vi "CreateSystemReference.vi"(8 "error in (no error)":errorcluster, 9 "Pane":refnum<vi>, 10 "ThisVIReference":refnum<vi>) -> (0 "error out":errorcluster, 1 "CommandQueueOut":refnum<queue>, 2 "DataNotifierOut":refnum<notifier>, 3 "ControlValueChangeEventRef":refnum<event-registration>)   [LabVIEW 2013]
uses:
  SystemData.lvclass/SystemData.lvclass
  RootCommand.lvclass/RootCommand.lvclass
  <vilib>/Utility/miscctls.llb/LVPointTypeDef.ctl
  Initialize.lvclass/Initialize.lvclass
  SystemData.lvclass/SystemData.lvclass/SystemData.ctl
  Generator.lvclass/Generator.lvclass
panel:
  # "建立系統運行參考"
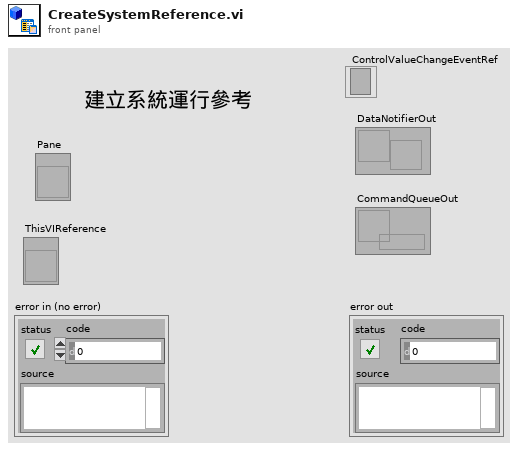
[diagram p1: front panel]
types:
  T1 = typedef "LVPointTypeDef.ctl" = cluster{"Horizontal":i16, "Vertical":i16}
  T2 = typedef "SystemData.lvclass/SystemDataTypeDefine.ctl" = cluster{"ThisVIParameter":cluster{"ThisVIPath":path, "ThisVIReference":refnum<vi>, "AllControlReference":refnum<vi>[]}, "GeneratorParameter":cluster{"Frequency":dbl, "Amplitude":dbl}, "WaveformBuffer":waveform(dbl), "SourceSelect":u16, "GeneratorClassArray":refnum<class "Generator.lvclass">[]}
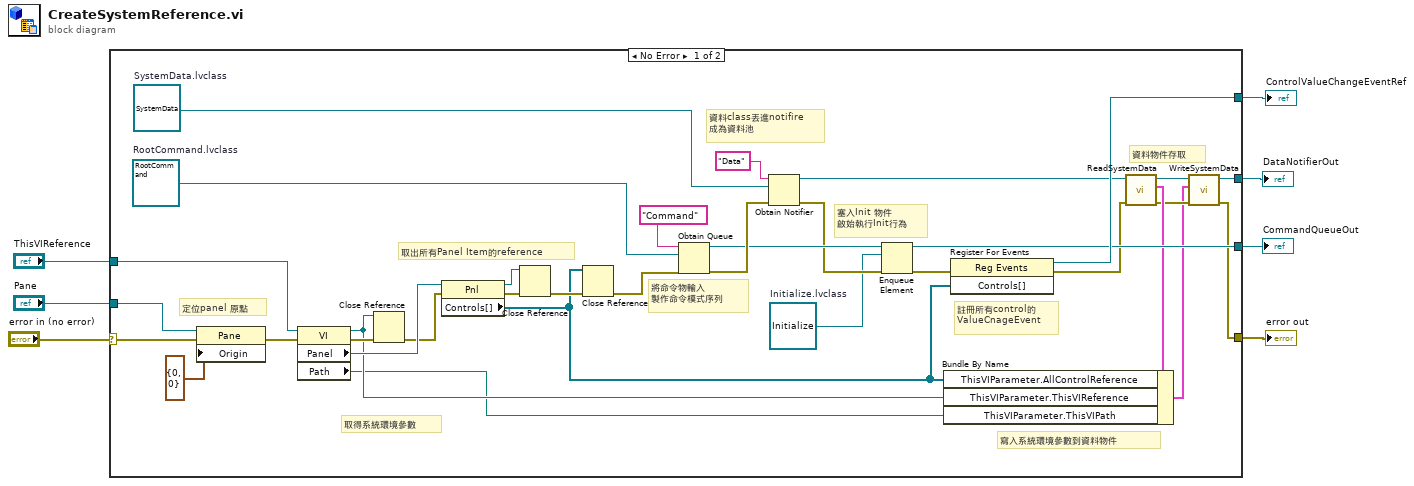
[diagram p0: block diagram]
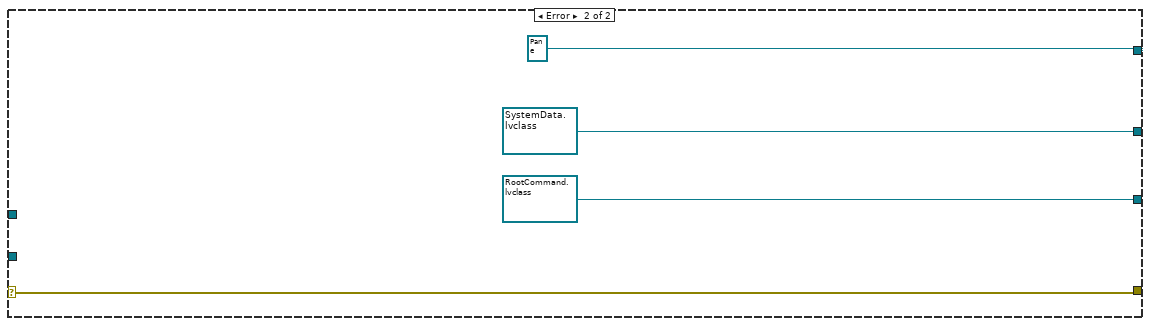
[diagram p2: hidden frame]
diagram:
  n1 = case shown="No Error" "error in (no error)" {
    selector: "error in (no error)" -> [w16 w45]
    tunnel: [w41 refnum<event-registration> refnum ("Event Registration Refnum")] -> w7
    tunnel: [w27 refnum<notifier> refnum ("DataNotifierOut")] -> w2
    tunnel: [w36 refnum<queue> refnum ("queue out")] -> w1
    tunnel: [w23 w45] -> w6
    tunnel: "ThisVIReference" -> [w29 _]
    tunnel: "Pane" -> [w15 _]
    frame No Error {
      w10 = refnum<class "Initialize.lvclass"> refnum  # Initialize.lvclass
      w20 = refnum<class "SystemData.lvclass"> refnum  # SystemData.lvclass
      w19 = refnum<class "RootCommand.lvclass"> refnum  # RootCommand.lvclass
      # "定位panel 原點"
      # "資料物件存取"
      # "塞入Init 物件\n啟始執行Init行為"
      # "取出所有Panel Item的reference"
      # "取得系統環境參數"
      # "寫入系統環境參數到資料物件"
      # "註冊所有control的\nValueCnageEvent"
      # "資料class丟進notifire\n成為資料池"
      # "將命令物輸入\n製作命令模式序列"
      n2 = property class="Pane"(reference=w15, error in=w16, "Origin"=T1 {"Horizontal"=0, "Vertical"=0}) -> (error out=w17:errorcluster)  [unwired: 1 out]
      n3 = property class="VI"(reference=w29, error in=w17) -> (reference out=w22:refnum<vi>, error out=w30:errorcluster, "Panel"=w31:refnum<vi>, "Path"=w21:path)
      n4 = Close Reference(reference=w22, error in (no error)=w30) -> (error out=w18:errorcluster)
      n5 = property class="Pnl"(reference=w31, error in=w18) -> (reference out=w33:refnum<vi>, error out=w32:errorcluster, "Controls[]"=w8:refnum<vi>[])
      n6 = Close Reference(reference=w33, error in (no error)=w32) -> (error out=w9:errorcluster)
      n7 = Close Reference(reference=w8, error in (no error)=w9) -> (error out=w11:errorcluster)
      n8 = Obtain Queue(name (unnamed)="Command", element data type=w19, error in (no error)=w11) -> (queue out=w37:refnum<queue>, error out=w40:errorcluster)  [unwired: 2 in, 1 out]
      n9 = Obtain Notifier(name (unnamed)="Data", notification data type=w20, error in (no error)=w40) -> (notifier out=w12:refnum<notifier>, error out=w35:errorcluster)  [unwired: 1 in, 1 out]
      n10 = Enqueue Element(queue=w37, element=w10, error in (no error)=w35) -> (queue out=w36:refnum<queue>, error out=w34:errorcluster)  [unwired: 1 in, 1 out]
      n11 = register-events(error in=w34, w8) -> (reference out=w41:refnum<event-registration>, error out=w26:errorcluster)  [unwired: 1 in]
      n12 = call "ReadSystemData.vi"("error in (no error)"=w26, "DataNotifierIn"=w12) -> ("error out"=w24:errorcluster, "SystemData"=w25:T2, "DataNotifierIn"=w28:refnum<notifier>)  [unwired: 7 in]
      n13 = Bundle By Name(cluster=w25, "ThisVIParameter.AllControlReference"=w8, "ThisVIParameter.ThisVIReference"=w22, "ThisVIParameter.ThisVIPath"=w21) -> (w13:T2)
      n14 = call "WriteSystemData.vi"("error in (no error)"=w24, "SystemData"=w13, "DataNotifierIn"=w28) -> ("error out"=w23:errorcluster, "DataNotifierOut"=w27:refnum<notifier>)  [unwired: 7 in]
    }
    frame Error {
    }
  }
  "error out" <- w6
  "ControlValueChangeEventRef" <- w7
  "DataNotifierOut" <- w2
  "CommandQueueOut" <- w1
